vi "4Pi Capture Write DM.vi"(6 "Next mode?":bool, 7 "Amp step size":dbl, 8 "Current Amp Step":u16, 9 "Current Mirror Mode":u16, 10 "Mirror Mode":u16[](array[numeric]), 11 "No. Amp steps":u16) -> ()   [LabVIEW 2016]
uses:
  4Pi Dual DM Control/4Pi Dual DM - Controls/4Pi Dual DM - Standard Action.ctl
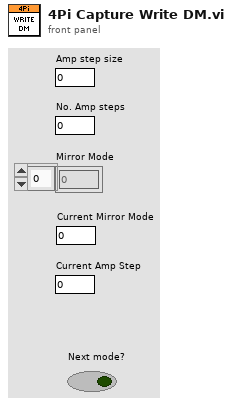
[diagram p1: front panel]
types:
  T1 = typedef "4Pi Dual DM - Standard Action.ctl" = enum16{"Read", "Write"}
  T2 = typedef "4Pi Dual DM - Mirror Modes DUAL.ctl" = cluster{"Mode":string, "Amplitude":dbl}[][]
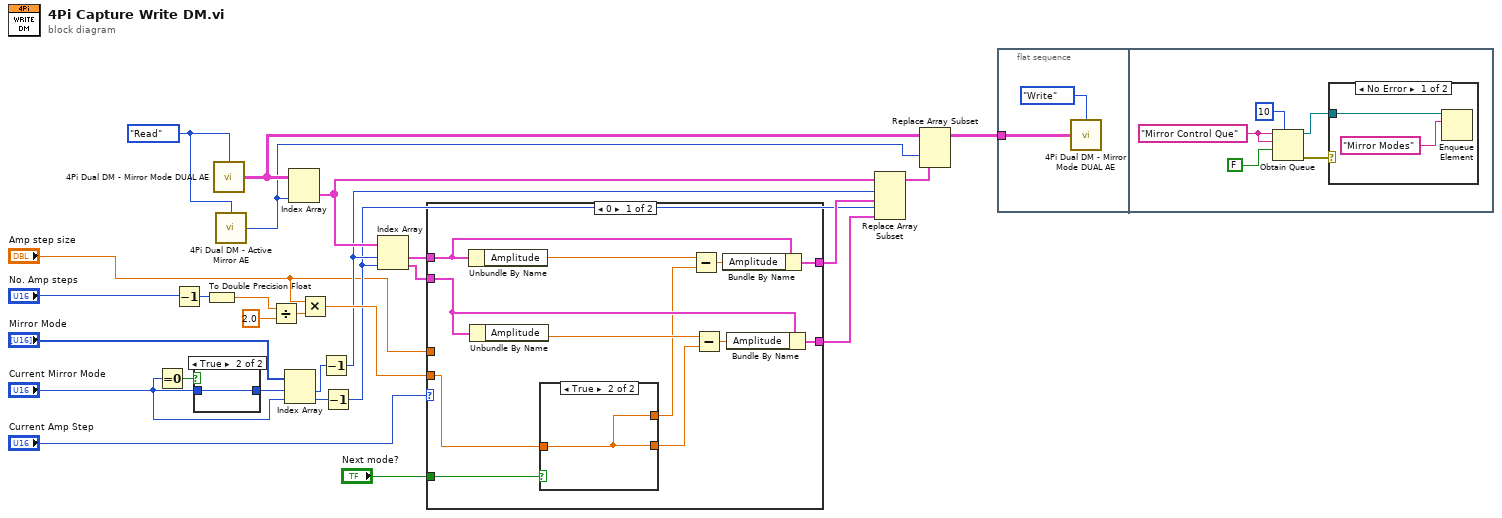
[diagram p0: block diagram]
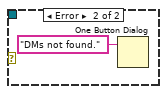
[diagram p2: hidden frame]
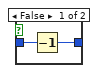
[diagram p3: hidden frame]
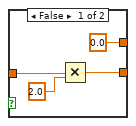
[diagram p4: hidden frame]
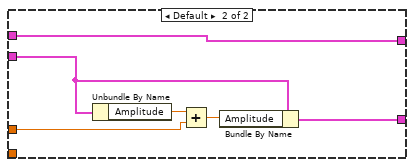
[diagram p5: hidden frame]
diagram:
  w27 = 4Pi_Dual_DM_-_Standard_Action."Read" ("Action")
  n1 = Equal To 0?(x="Current Mirror Mode") -> (x = 0?=w12:bool)
  n2 = Decrement(x="No. Amp steps") -> (x-1=w15:u16)
  n3 = case shown="True" w12 {
    tunnel: [w29 w30] -> w22
    tunnel: "Current Mirror Mode" -> [w28 w30]
    frame False {
      n4 = Decrement(x=w28) -> (x-1=w29:u16)
    }
    frame True {
    }
  }
  n5 = To Double Precision Float(number=w15) -> (double precision float=w14:dbl)
  n6 = call "4Pi Dual DM - Mirror Mode DUAL AE.vi"("Action"=w27) -> ("Mirror Modes Out"=w26:T2)  [unwired: 14 in]
  n7 = call "4Pi Dual DM - Active Mirror AE.vi"("Action"=w27) -> ("Active Mirror"=w23:i32)  [unwired: 14 in]
  n8 = Divide(x=w14, y=2.0) -> (x/y=w17:dbl)
  n9 = Index Array(array="Mirror Mode", index #1=w22, index #2="Current Mirror Mode") -> (element #1=w10:u16, element #2=w9:u16)
  n10 = Index Array(array=w26, index (col)=w23) -> (element=w24:cluster{"Mode":string, "Amplitude":dbl}[])  [unwired: 1 in]
  n11 = Multiply(x="Amp step size", y=w17) -> (x*y=w13:dbl)
  n12 = Decrement(x=w10) -> (x-1=w11:u16)
  n13 = Decrement(x=w9) -> (x-1=w8:u16)
  n14 = Index Array(array=w24, index #1=w11, index #2=w8) -> (element #1=w20:cluster{"Mode":string, "Amplitude":dbl}, element #2=w21:cluster{"Mode":string, "Amplitude":dbl})
  n15 = case shown="0" "Current Amp Step" {
    tunnel: w21 -> [w41 w53]
    tunnel: "Amp step size" -> [_ w51]
    tunnel: [w39 w49] -> w18
    tunnel: w20 -> [w37 w48]
    tunnel: [w35 w48] -> w19
    tunnel: w13 -> [w34 _]
    tunnel: "Next mode?" -> [w33 _]
    frame 0 {
      n16 = Unbundle By Name(w37) -> ("Amplitude"=w38:dbl)
      n17 = Unbundle By Name(w41) -> ("Amplitude"=w42:dbl)
      n18 = case shown="True" w33 {
        tunnel: w34 -> [w46 w47]
        tunnel: [w44 w47] -> w32
        tunnel: [0.0 w47] -> w31
        frame False {
          n19 = Multiply(x=w46, y=2.0) -> (x*y=w44:dbl)
        }
        frame True {
        }
      }
      n20 = Subtract(x=w38, y=w31) -> (x-y=w36:dbl)
      n21 = Subtract(x=w42, y=w32) -> (x-y=w40:dbl)
      n22 = Bundle By Name(cluster=w37, "Amplitude"=w36) -> (w35:cluster{"Mode":string, "Amplitude":dbl})
      n23 = Bundle By Name(cluster=w41, "Amplitude"=w40) -> (w39:cluster{"Mode":string, "Amplitude":dbl})
    }
    frame Default {
      n24 = Unbundle By Name(w53) -> ("Amplitude"=w52:dbl)
      n25 = Add(x=w52, y=w51) -> (x+y=w50:dbl)
      n26 = Bundle By Name(cluster=w53, "Amplitude"=w50) -> (w49:cluster{"Mode":string, "Amplitude":dbl})
    }
  }
  n27 = Replace Array Subset(array=w24, new element #1=w19, index #1=w11, new element #2=w18, index #2=w8) -> (w25:cluster{"Mode":string, "Amplitude":dbl}[])
  n28 = Replace Array Subset(array=w26, new element=w25, index (col)=w23) -> (w7:T2)  [unwired: 1 in]
  n29 = flat-sequence {
    tunnel: w7 -> [w54]
    frame #0 {
      n30 = call "4Pi Dual DM - Mirror Mode DUAL AE.vi"("Action"=4Pi_Dual_DM_-_Standard_Action."Write", "Mirror Modes In"=w54) -> ()  [unwired: 13 in, 1 out]
    }
    frame #1 {
      w56 = "Mirror Control Que" ("name (unnamed)")
      n31 = Obtain Queue(max queue size (-1, unlimited)=10, name (unnamed)=w56, element data type=w56, create if not found? (T)=FALSE) -> (queue out=w60:refnum<queue>, error out=w59:errorcluster)  [unwired: 1 in, 1 out]
      n32 = case shown="No Error" w59 {
        tunnel: w60 -> [w61 _]
        frame No Error {
          n33 = Enqueue Element(queue=w61, element="Mirror Modes" ("name (unnamed)")) -> ()  [unwired: 2 in, 3 out]
        }
        frame Error {
          n34 = One Button Dialog(message="DMs not found.") -> ()  [unwired: 1 in, 1 out]
        }
      }
    }
  }
